vi "Measurement Logic.vi"() -> ()   [LabVIEW 2021, in "niScope EX Getting Started.lvlib"]
uses:
  niScope EX Getting Started.lvlib
  <vilib>/Plug-In SDKs/Measurements/Measure Call Context/Measure Call Context.lvclass
  <vilib>/Plug-In SDKs/Sessions/niScope/NI Session Management niScope.lvlib
  <vilib>/Plug-In SDKs/Clients/Session Management V1/Session Reservation/Session Reservation.lvclass
  4e8d0f78-792a-4020-9afa-03c2d49fbc62.vi
  Measurement Configuration.ctl
  Measurement Results.ctl
panel:
  out "measure call context out":refnum<class "Measure Call Context.lvclass">
  in  "measure call context in":refnum<class "Measure Call Context.lvclass">
  out "measurement results":T1
  in  "measurement configuration":T2={"Channel(s)"="Lorem ipsum dolor sit", "Simulate?"=TRUE, "resource name Pin"=""}
  out "error out":errorcluster
  in  "error in":errorcluster
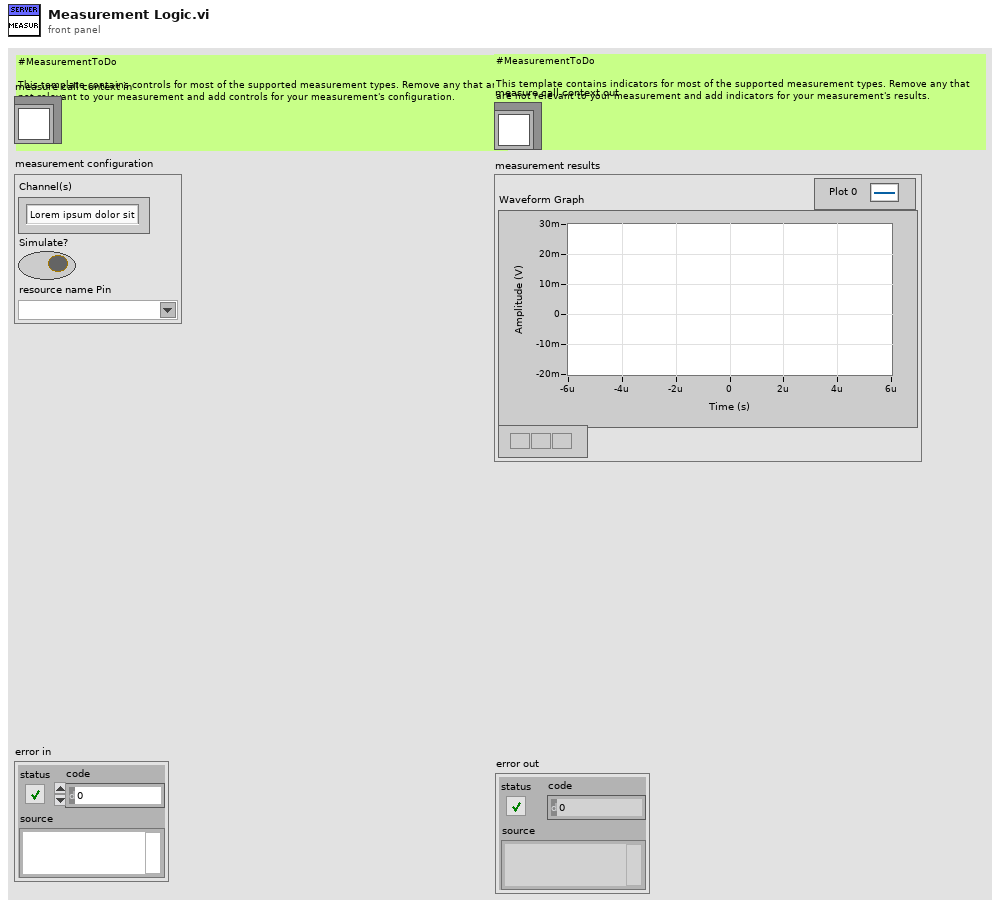
[diagram p1: front panel]
types:
  T1 = typedef "niScope EX Getting Started.lvlib/Measurement Results.ctl" = cluster{"Waveform Graph":cluster{"relativeInitialX":dbl, "xIncrement":dbl, "wfm":dbl[]}[]}
  T2 = typedef "niScope EX Getting Started.lvlib/Measurement Configuration.ctl" = cluster{"Channel(s)":string, "Simulate?":bool, "resource name Pin":string}
  T3 = typedef "NI Session Management niScope.lvlib/Connection with Session.ctl" = cluster{"connection":T4, "session":refnum<k15>}
  T4 = typedef "NI Session Management V1 Client.lvlib/Session Reservation.lvclass/Connection.ctl" = cluster{"pin or relay name":string, "site":i32, "instrument type id":string, "channel":string}
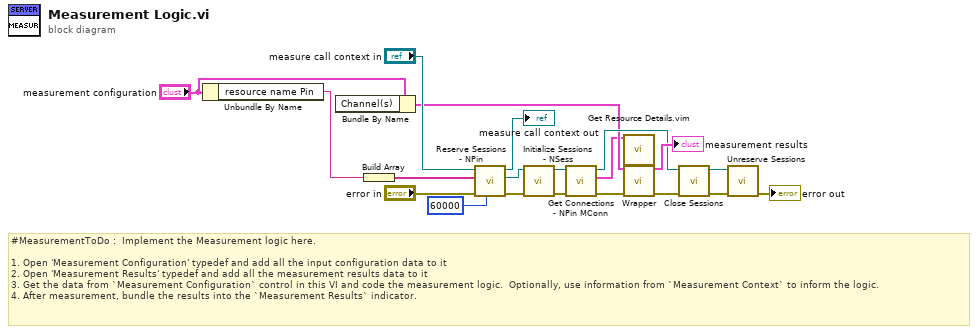
[diagram p0: block diagram]
diagram:
  # "#MeasurementToDo :  Implement the Measurement logic here.\n\n1. Open 'Measurement Configuration' typedef and add all the input configuration data to it\n2. Open 'Measurement Results' typedef and add all the measurement results data to it\n3. Get the data from `Measurement Configuration` control in this VI and code the measurement logic.  Optionally, use information from `Measurement Context` to inform the logic.\n4. After measurement, bundle the results into the `Measurement Results` indicator."
  n1 = Unbundle By Name("measurement configuration") -> ("resource name Pin"=w19:string)
  n2 = Bundle By Name(cluster="measurement configuration") -> (w2:T2)  [unwired: 1 in]
  n3 = Build Array(w19) -> (w15:string[])
  n4 = call <vilib>:"Reserve Sessions - NPin.vi"("timeout (ms)"=60000, "error in"="error in", "pin or relay names"=w15, "measurement context in"="measure call context in") -> ("error out"=w13:errorcluster, "session reservation out"=w12:refnum<class "Session Reservation.lvclass">, "measurement context out"=→"measure call context out":refnum<class "Measure Call Context.lvclass">)  [unwired: 5 in]
  n5 = call <vilib>:"Initialize Sessions - NSess.vi"("error in"=w13, "session reservation in"=w12) -> ("error out"=w11:errorcluster, "session reservation out"=w10:refnum<class "Session Reservation.lvclass">)  [unwired: 6 in, 2 out]
  n6 = call <vilib>:"Get Connections - NPin MConn.vi"("error in"=w11, "session reservation in"=w10) -> ("error out"=w8:errorcluster, "connections"=w1:T3[], "session reservation out"=w6:refnum<class "Session Reservation.lvclass">)  [unwired: 7 in]
  n7 = call "Get Resource Details.vim"("connections"=w1) -> ()  [unwired: 13 in, 2 out]
  n8 = call "Wrapper.vi"("measurement configuration"=w2, "error in"=w8) -> ("measurement results"=→"measurement results":T1, "error out"=w7:errorcluster)  [unwired: 12 in]
  n9 = call <vilib>:"Close Sessions.vi"("error in"=w7, "session reservation in"=w6) -> ("error out"=w4:errorcluster, "session reservation out"=w3:refnum<class "Session Reservation.lvclass">)  [unwired: 8 in]
  n10 = call <vilib>:"Unreserve Sessions.vi"("error in"=w4, "session reservation in"=w3) -> ("error out"=→"error out":errorcluster)  [unwired: 9 in]
